vi "Sine Pattern.vi"(2 "cycles":dbl=1.0 format="%0.2f", 3 "phase(degrees)":dbl format="%0.2f", 4 "amplitude":dbl=1.0 format="%0.2f", 5 "samples":i32=128) -> (0 "error":i32, 1 "Sinusoidal Pattern":dbl[](array[numeric]))   [LabVIEW 2017, in "NI_AALBase.lvlib"]
doc: "Generates an array containing a sinusoidal pattern."
uses:
  <vilib>/Analysis/NI_AALBase.lvlib
  <resource>/lvanlys.dll
panel:
  # "Sine Pattern"
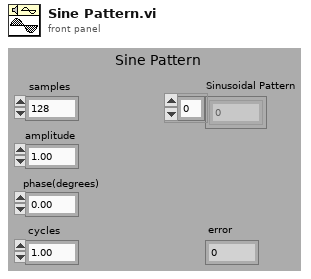
[diagram p1: front panel]
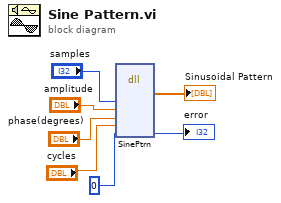
[diagram p0: block diagram]
diagram:
  n1 = dll-call lib="e:/builds/penguin/labview/branches/2017/dev/dist/resource/lvanlys.*" fn="SinePtrn"("samples"="samples", "amplitude"="amplitude", "phase(degrees)"="phase(degrees)", "cycles"="cycles", 0) -> ("Sinusoidal Pattern"=→"Sinusoidal Pattern":dbl[], →"error":i32)  [unwired: 9 in, 2 out]
